vi "waveform_stats.vi"(8 "Waveform Data":waveform(dbl)[](graph)=[{"t0"=timestamp(1.749999999999907e-07 s since 1904-01-01), "dt"=1e-10, "Y"=array[1000 elements]}]) -> (3 "stats":T1[](array[typedef]))   [LabVIEW 2015, in "oskar_tools.lvlib"]
uses:
  oskar_tools.lvlib
  acquisition/fake_oscilloscope/osc_stats.ctl
  <vilib>/Analysis/NI_AALBase.lvlib
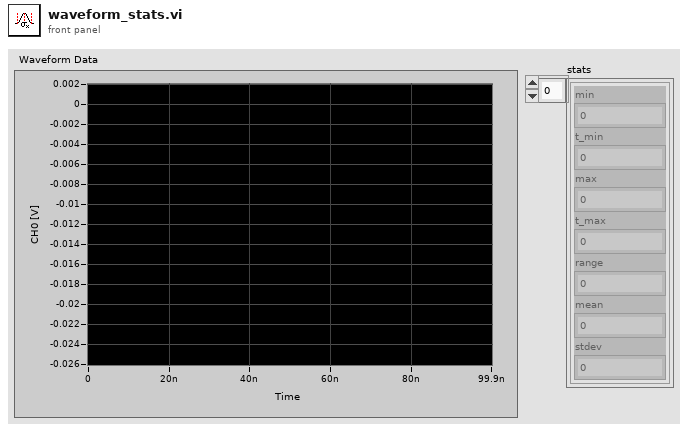
[diagram p1: front panel]
types:
  T1 = typedef "osc_stats.ctl" = cluster{"min":dbl, "t_min":dbl, "max":dbl, "t_max":dbl, "range":dbl, "mean":dbl, "stdev":dbl}
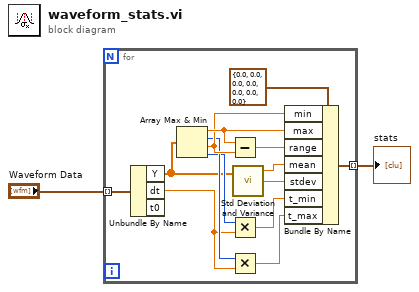
[diagram p0: block diagram]
diagram:
  n1 = for {
    tunnel: "Waveform Data" -> [w16] mode=indexing
    tunnel: [w10] -> w1 mode=indexing
    n2 = Unbundle By Name(w16) -> ("Y"=w3:dbl[], "dt"=w6:dbl)  [unwired: 1 out]
    n3 = Array Max & Min(array=w3) -> (max value=w15:dbl, max index (indices)=w9:i32, min value=w14:dbl, min index (indices)=w7:i32)
    n4 = Subtract(x=w15, y=w14) -> (x-y=w13:dbl)
    n5 = Multiply(x=w7, y=w6) -> (x*y=w5:dbl)
    n6 = Multiply(x=w9, y=w6) -> (x*y=w8:dbl)
    n7 = call <vilib>:"Std Deviation and Variance.vi"("X"=w3) -> ("mean"=w12:dbl, "standard deviation"=w11:dbl)  [unwired: 1 in, 1 out]
    n8 = Bundle By Name(cluster=T1 {"min"=0.0, "t_min"=0.0, "max"=0.0, "t_max"=0.0, "range"=0.0, "mean"=0.0, "stdev"=0.0} ("info"), "min"=w14, "max"=w15, "range"=w13, "mean"=w12, "stdev"=w11, "t_min"=w5, "t_max"=w8) -> (w10:T1)
  }
  "stats" <- w1
